vi "Game_RandomlyPlaceItems.vi"   [LabVIEW 2018]
uses:
  <vilib>/rvi/Emulation/niFpgaGetClockAttributes.vi
  <vilib>/rvi/Emulation/niFpgaSctlEmulationGetInTimedLoop.vi
  <vilib>/rvi/Emulation/niFpgaEmulationReportErrorSimple.vi
  Control/Global_GameOver.vi
  <vilib>/rvi/Emulation/niFpgaCriticalErrorInLSC.vi
  <vilib>/rvi/Memory/Memory_Emulation/nirvimemoryFastEmulation.vi
  <vilib>/rvi/Memory/Memory_Emulation/nirvimemoryEmulation.vi
  <vilib>/rvi/Emulation/niFpgaEmulationIsFPGAContextNoSignature.vi
  <vilib>/rvi/DataTransferAndStorage/Container/Common/niFpgaContainerGetUniqueNameForEmu.vi
  <vilib>/rvi/Emulation/niFpgaProcessEmulError.vi
  <vilib>/rvi/errors/nirviReportUnexpectedCaseInternalError (U32).vi
  <vilib>/rvi/DataTransferAndStorage/Container/XNode/niFpgaContainer.xnode
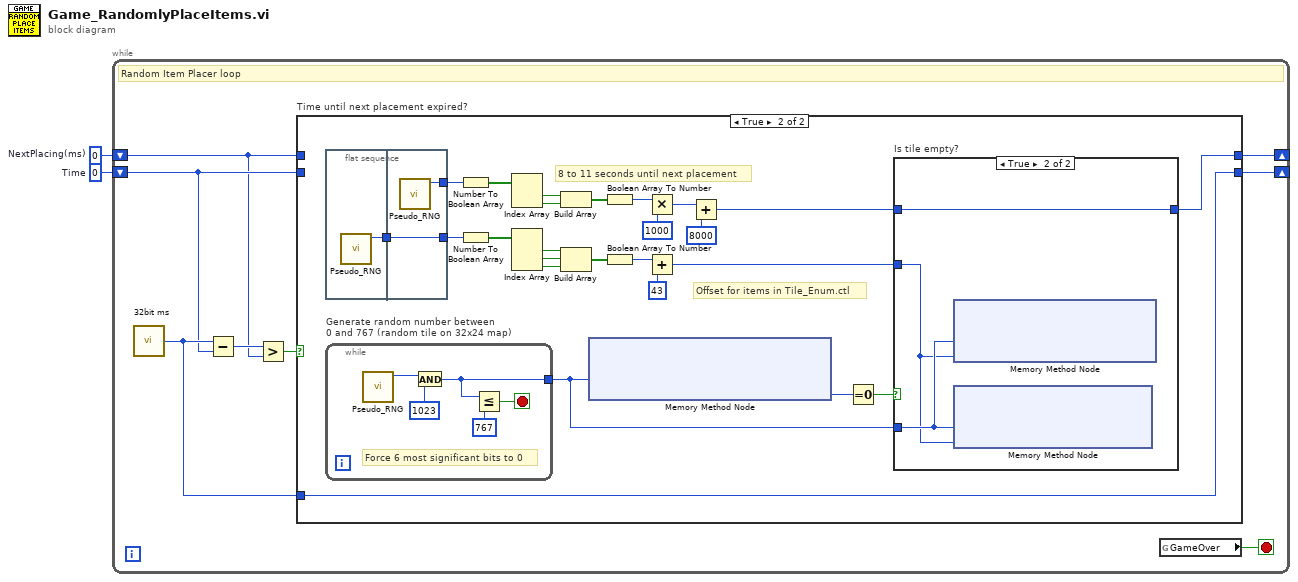
[diagram p0: block diagram]
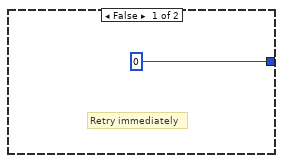
[diagram p3: hidden frame]
diagram:
  w1 = u32 0  # Time
  w2 = u32 0  # NextPlacing(ms)
  n1 = while {
    shift-right: [w6] -> _
    shift-left: w1 -> [w4]
    shift-right: [w8] -> _
    shift-left: w2 -> [w3]
    stop <- w10 stop-if-true
    # "Random Item Placer loop"
    n2 = call "32bit ms"() -> ("Tick Count(mSec)"=w5:u32)
    n3 = Subtract(x=w5, y=w4) -> (x-y=w9:u32)
    n4 = Greater?(x=w9, y=w3) -> (0:w7:bool)
    n5 = case "Time until next placement expired?" shown="True" w7 {
      tunnel: [w12 w37] -> w8
      tunnel: w3 -> [w12 _]
      tunnel: w4 -> [w11 _]
      tunnel: [w11 w36] -> w6
      tunnel: w5 -> [_ w36]
      frame False {
      }
      frame True {
        # "Offset for items in Tile_Enum.ctl"
        # "8 to 11 seconds until next placement"
        n6 = flat-sequence {
          tunnel: [w38] -> w13
          tunnel: [w40] -> w15
          tunnel: [w39] -> w14
          tunnel: w13 -> [w39]
          frame #0 {
            n7 = call "Pseudo_RNG.vi"() -> ("pseudo random value"=w38:u16)  [unwired: 11 in]
          }
          frame #1 {
            n8 = call "Pseudo_RNG.vi"() -> ("pseudo random value"=w40:u16)  [unwired: 11 in]
          }
        }
        n9 = while "Generate random number between\n0 and 767 (random tile on 32x24 map)" {
          tunnel: [w41] -> w33
          stop <- w42 stop-if-true
          # "Force 6 most significant bits to 0"
          n10 = call "Pseudo_RNG.vi"() -> ("pseudo random value"=w44:u16)  [unwired: 11 in]
          n11 = And(x=w44, y=u16 1023) -> (x .and. y?=w41:u16)
          n12 = Less Or Equal?(x=w41, y=u16 767) -> (x <= y?=w42:bool)
        }
        n13 = Number To Boolean Array(number=w15) -> (Boolean array=w27:bool[])
        n14 = Number To Boolean Array(number=w14) -> (Boolean array=w18:bool[])
        n15 = Index Array(array=w27) -> (element #1=w28:bool, element #2=w29:bool)  [unwired: 2 in]
        n16 = Index Array(array=w18) -> (element #1=w21:bool, element #2=w22:bool, element #3=w19:bool)  [unwired: 3 in]
        n17 = Build Array(w28, w29) -> (w25:bool[])
        n18 = Build Array(w21, w22, w19) -> (w20:bool[])
        n19 = xnode ("Memory Method Node")("Address"=w33) -> ("Data"=w35:u8)  [unwired: 1 in, 1 out]
        n20 = Boolean Array To Number(Boolean array=w25) -> (number=w32:u32)
        n21 = Boolean Array To Number(Boolean array=w20) -> (number=w23:u8)
        n22 = Multiply(x=w32, y=u32 1000) -> (x*y=w30:u32)
        n23 = Add(x=w23, y=u8 43) -> (x+y=w16:u8)
        n24 = Add(x=w30, y=u32 8000) -> (x+y=w17:u32)
        n25 = Equal To 0?(x=w35) -> (x = 0?=w34:bool)
        n26 = case "Is tile empty?" shown="True" w34 {
          tunnel: [u32 0 w48] -> w37
          tunnel: w33 -> [_ w49]
          tunnel: w17 -> [_ w48]
          tunnel: w16 -> [_ w47]
          frame False {
            # "Retry immediately"
          }
          frame True {
            n27 = xnode ("Memory Method Node")("Address"=w49, "Data"=w47) -> ()  [unwired: 1 in, 1 out]
            n28 = xnode ("Memory Method Node")("Address"=w49, "Data"=w47) -> ()  [unwired: 1 in, 1 out]
          }
        }
      }
    }
    n29 = global read "Global_GameOver.vi" "GameOver"() -> (w10:bool)
  }
